vi "InsertIntoCircularBuffer-Numbers.vi"(8 "NewElements":dbl[](array[numeric]), 10 "StartIndex":dbl, 11 "Buffer":dbl[](array[numeric])) -> (1 "New Start Index":dbl, 2 "UpdatedBuffer":dbl[](array[numeric]))   [LabVIEW 2016]
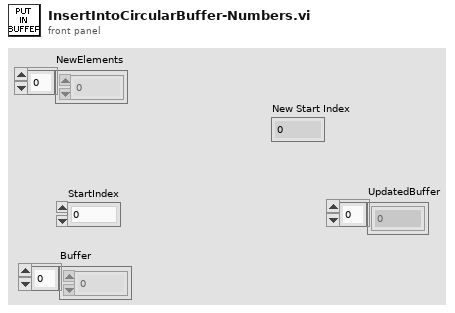
[diagram p1: front panel]
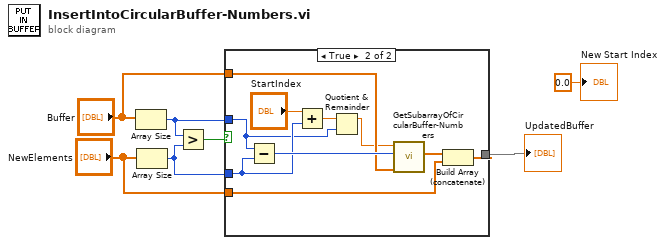
[diagram p0: block diagram]
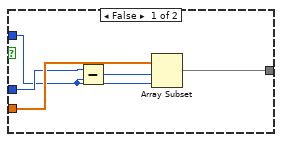
[diagram p2: hidden frame]
diagram:
  n1 = Array Size(array="Buffer") -> (size(s)=w5:i32)
  n2 = Array Size(array="NewElements") -> (size(s)=w4:i32)
  n3 = Greater?(x=w5, y=w4) -> (0:w6:bool)
  n4 = case shown="True" w6 {
    tunnel: [w11 w22] -> w7
    tunnel: w5 -> [w9 w15]
    tunnel: w4 -> [w10 w17]
    tunnel: "Buffer" -> [_ w19]
    tunnel: "NewElements" -> [w12 w13]
    frame False {
      n5 = Subtract(x=w10, y=w9) -> (x-y=w8:i32)
      n6 = Array Subset(array=w12, index=w8, length=w9) -> (w11:dbl[])
    }
    frame True {
      n7 = Subtract(x=w15, y=w17) -> (x-y=w21:i32)
      n8 = Add(x="StartIndex", y=w17) -> (x+y=w16:dbl)
      n9 = Quotient & Remainder(x=w16, y=w15) -> (x-y*floor(x/y)=w14:dbl)  [unwired: 1 out]
      n10 = call "GetSubarrayOfCircularBuffer-Numbers.vi"("buffer"=w19, "subset size"=w21, "start index"=w14) -> ("subarray"=w20:dbl[])  [unwired: 8 in]
      n11 = Build Array (concatenate)(w20, w13) -> (w22:dbl[])
    }
  }
  "UpdatedBuffer" <- w7
  "New Start Index" <- 0.0 ("New Start Index")
